vi "CFocus.vi"() -> ()   [LabVIEW 2012]
uses:
  Madlib.dll
panel:
  in  "Read Rate":bool=TRUE
  in  "Stream Rate":i32(slide)=100 min=100 max=1000 step=1 scale=100.0..1000.0 scale format="%#.0f"
  out "resetProgress":u8(slide) scale=0.0..100.0
  in  "resetEncoder":bool
  out "Graph":T1(graph)
  in  "C-Focus":bool
  out "MCL_Error":i32
  out "Tab Control":enum32{"Position Control", "C-Focus Control"}(tab)
  in  "Position":dbl
  in  "Command":bool
  in  "Start":dbl min=0.0
  in  "End":dbl min=0.0
  in  "# of Steps":dbl=1.0 min=1.0
  in  "Dwell Time":u32
  out "Calculated Step Size":dbl
  in  "Z-Stack":bool
  in  "Relative position\nchange from current":dbl step=0.005
  in  "CF command":bool
  out "Enabled at (ADC)":dbl format="%#.4f"
  in  "Z-Stack with C-Focus":bool
  in  "Dwell Time 2":u32
  in  "# of Steps 2":dbl=1.0 min=1.0
  out "End 2":dbl min=0.0 format="%#.4f"
  out "Start 2":dbl min=0.0 format="%#.4f"
  in  "Step Size":dbl step=0.005
  out "EncoderStart":dbl
  out "Error":i32
  in  "EndVI":bool
  out "Mode Bar":enum32{"Standard", "Cfocus"}(tab)
  # "Enable/Disable Constant Focus"
  # "Stream\nRate"
  # "Read\nRate"
  # "fast"
  # "slow"
  # "fast"
  # "slow"
  # "Positioning"
  # "um"
  # "Z-Stack"
  # "um"
  # "um"
  # "ms"
  # "um"
  # "Position Info"
  # "um"
  # "C-Focus Positioning"
  # "um"
  # "C-Focus Z-Stack"
  # "um"
  # "ms"
  # "um"
  # "um"
  # "Standard Position Control"
  # "Constant Focus Mode Enabled"
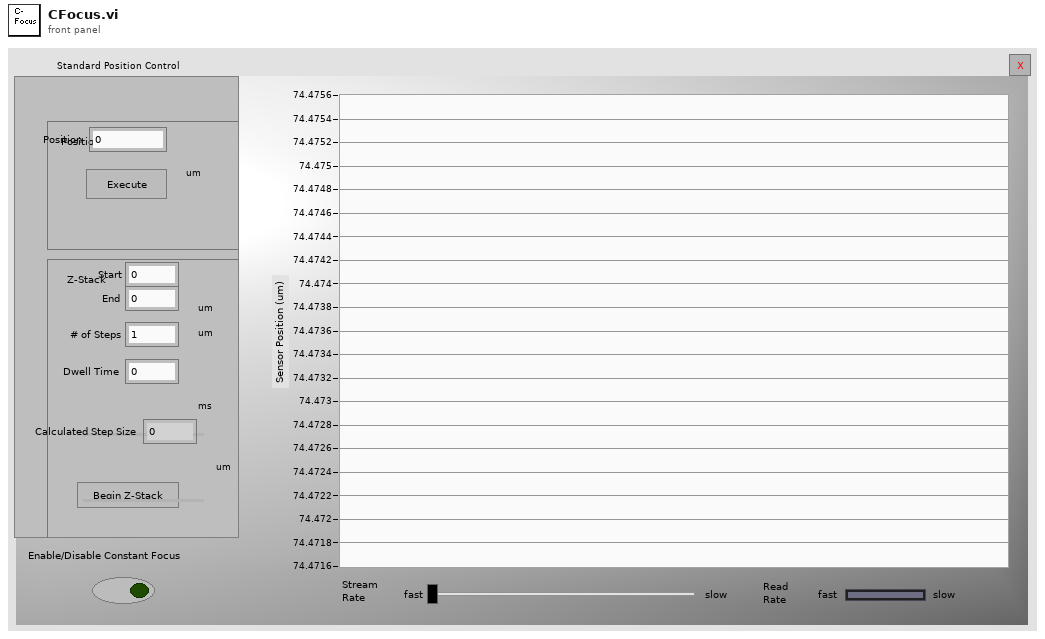
[diagram p1: front panel]
types:
  T1 = cluster{"Encoder Set":dbl, "Encoder Set":dbl, dbl[][]}
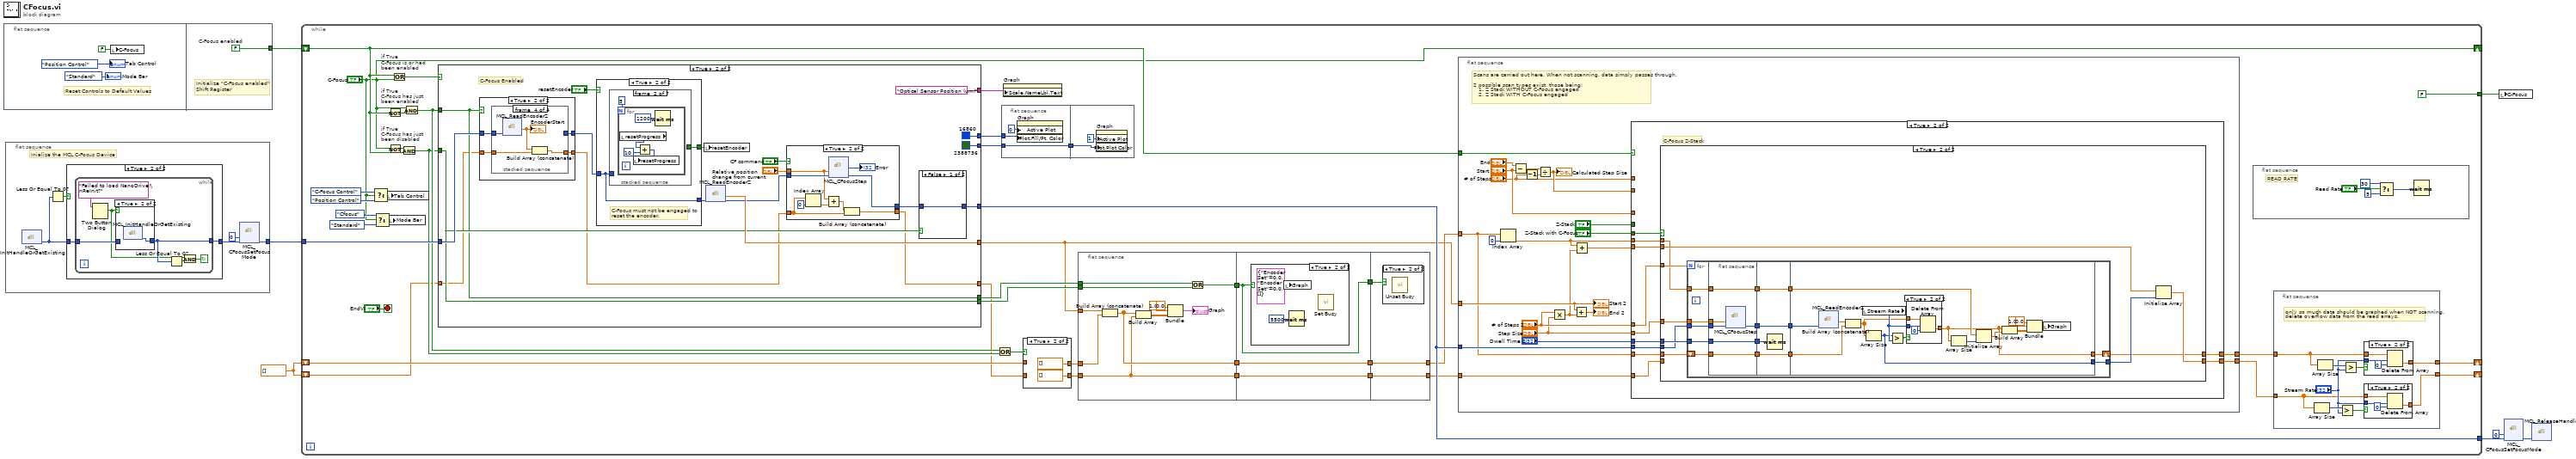
[diagram p0: block diagram]
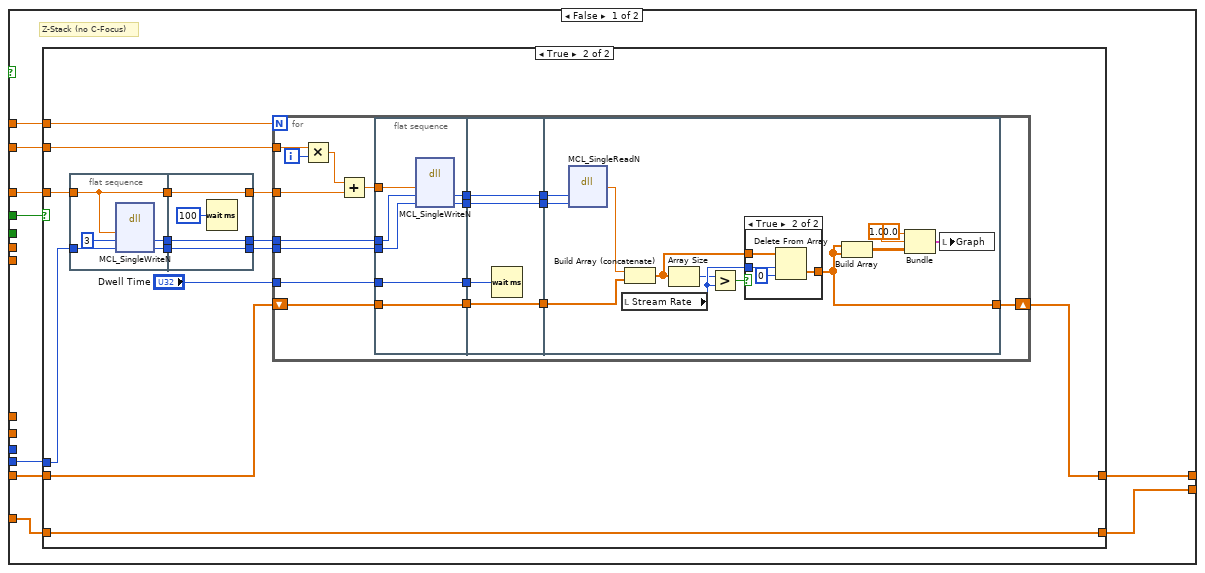
[diagram p4: hidden frame]
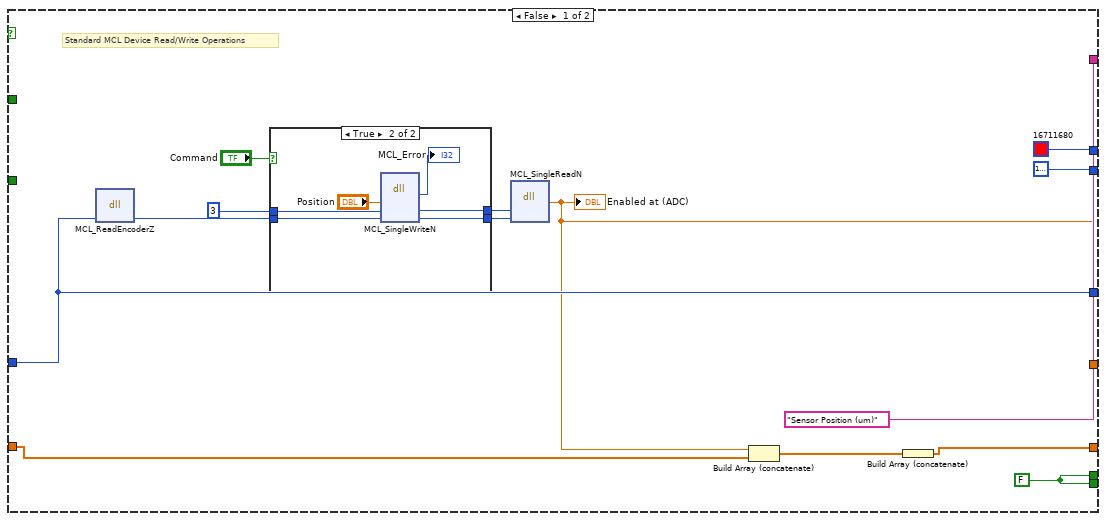
[diagram p14: hidden frame]
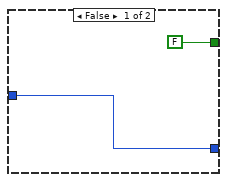
[diagram p16: hidden frame]
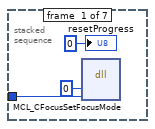
[diagram p17: hidden frame]
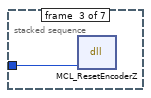
[diagram p18: hidden frame]
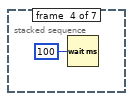
[diagram p19: hidden frame]
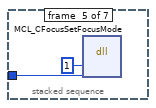
[diagram p20: hidden frame]
diagram:
  w1 = dbl[] []
  n1 = flat-sequence {
    tunnel: [w11] -> w2
    frame #0 {
      # "Reset Controls to Default Values"
      n2 = local write "C-Focus"(FALSE ("C-Focus")) -> ()
      "Tab Control" <- enum32{"Position Control", "C-Focus Control"}."Position Control" ("Tab Control")
      "Mode Bar" <- enum32{"Standard", "Cfocus"}."Standard" ("Mode Bar")
    }
    frame #1 {
      w11 = FALSE  # C-Focus enabled
      # "Initialize \"C-Focus enabled\"\nShift Register"
    }
  }
  n3 = flat-sequence {
    tunnel: [w12] -> w6
    frame #0 {
      # "Inialize the MCL C-Focus Device"
      n4 = dll-call lib="C:/Users/Labview/Desktop/SRR/Madlib_x64/Labview Examples/Madlib.dll" fn="MCL_InitHandleOrGetExisting"() -> ("return type"=w15:i32)  [unwired: 3 in, 2 out]
      n5 = Less Or Equal To 0?(x=w15) -> (x <= 0?=w16:bool)
      n6 = case shown="True" w16 {
        tunnel: w15 -> [w17 w19]
        tunnel: [w17 w18] -> w13
        frame False {
        }
        frame True {
          n7 = while {
            tunnel: w19 -> [w24]
            tunnel: [w22] -> w18
            stop <- w21 continue-if-true
            n8 = Two Button Dialog(message="Failed to load NanoDrive!\nReInit?") -> (T button?=w20:bool)  [unwired: 2 out]
            n9 = case shown="True" w20 {
              tunnel: w24 -> [w26 _]
              tunnel: [w26 w27] -> w22
              frame False {
              }
              frame True {
                n10 = dll-call lib="C:/Users/Labview/Desktop/SRR/Madlib_x64/Labview Examples/Madlib.dll" fn="MCL_InitHandleOrGetExisting"() -> ("return type"=w27:i32)  [unwired: 3 in, 2 out]
              }
            }
            n11 = Less Or Equal To 0?(x=w22) -> (x <= 0?=w23:bool)
            n12 = And(x=w20, y=w23) -> (x .and. y?=w21:bool)
          }
        }
      }
      n13 = dll-call lib="C:/Users/Labview/Desktop/SRR/Madlib_x64/Labview Examples/Madlib.dll" fn="MCL_CFocusSetFocusMode" ("MADLib.dll:MCL_ReadEncoderZ")("C-Focus Enable"=i16 0, "handle"=w13) -> ("handle"=w12:i32)  [unwired: 4 in, 3 out]
    }
  }
  n14 = while {
    tunnel: [w66] -> w4
    tunnel: w6 -> [w68]
    shift-right: ["C-Focus"] -> _
    shift-left: w2 -> [w64]
    tunnel: [FALSE ("C-Focus")] -> w7
    shift-right: [w42] -> _
    shift-left: w1 -> [w52]
    shift-right: [w41] -> _
    shift-left: w1 -> [w46]
    stop <- "EndVI" stop-if-true
    # "if True\nC-Focus is or had been enabled"
    # "if True\nC-Focus has just\nbeen disabled"
    # "if True\nC-Focus has just\nbeen enabled"
    n15 = Select(t=enum32{"Position Control", "C-Focus Control"}."C-Focus Control" ("Tab Control"), s="C-Focus", f=enum32{"Position Control", "C-Focus Control"}."Position Control" ("Tab Control")) -> (s? t:f=w59:enum32{"Position Control", "C-Focus Control"})
    n16 = Select(t=enum32{"Standard", "Cfocus"}."Cfocus" ("Mode Bar"), s="C-Focus", f=enum32{"Standard", "Cfocus"}."Standard" ("Mode Bar")) -> (s? t:f=w37:enum32{"Standard", "Cfocus"})
    n17 = local write "Tab Control"(w59) -> ()
    n18 = Not(x=w64) -> (.not. x?=w63:bool)
    n19 = Not(x="C-Focus") -> (.not. x?=w62:bool)
    n20 = local write "Mode Bar"(w37) -> ()
    n21 = Or(x=w64, y="C-Focus") -> (x .or. y?=w65:bool)
    n22 = And(x=w62, y=w64) -> (x .and. y?=w47:bool)
    n23 = And(x="C-Focus", y=w63) -> (x .and. y?=w49:bool)
    n24 = case shown="True" w65 {
      tunnel: [w300 w331] -> w66
      tunnel: w68 -> [w300 w328]
      tunnel: w49 -> [_ w317]
      tunnel: w47 -> [_ w318]
      tunnel: [w295 w329] -> w28
      tunnel: [u32 16711680 u32 16860] -> w54
      tunnel: ["Sensor Position (um)" ("Y Scale.Unit Label.Text") "Optical Sensor Position (um)" ("Y Scale.Unit Label.Text")] -> w53
      tunnel: [w297 w318] -> w57
      tunnel: [w297 w317] -> w56
      tunnel: w46 -> [w291 w315]
      tunnel: [w294 w316] -> w45
      tunnel: [u32 16777216 u32 2388736] -> w43
      frame False {
        w297 = FALSE
        # "Standard MCL Device Read/Write Operations"
        n25 = dll-call lib="C:/Users/Labview/Desktop/SRR/Madlib_x64/Labview Examples/Madlib.dll" fn="MCL_ReadEncoderZ"("handle"=w300) -> ("handle"=w296:i32)  [unwired: 3 in, 3 out]
        n26 = case shown="True" "Command" {
          tunnel: w296 -> [w306 w312]
          tunnel: [w306 w311] -> w304
          tunnel: [w305 w310] -> w303
          tunnel: 3 ("axis") -> [w305 w308]
          frame False {
          }
          frame True {
            n27 = dll-call lib="C:/Users/Labview/Desktop/SRR/Madlib_x64/Labview Examples/Madlib.dll" fn="MCL_SingleWriteN"("Position"="Position", "axis"=w308, "handle"=w312) -> ("MCL_Error"=→"MCL_Error":i32, "axis"=w310:i32, "handle"=w311:i32)  [unwired: 4 in, 2 out]
          }
        }
        n28 = dll-call lib="C:/Users/Labview/Desktop/SRR/Madlib_x64/Labview Examples/Madlib.dll" fn="MCL_SingleReadN"("axis"=w303, "handle"=w304) -> ("Position Read"=w295:dbl)  [unwired: 5 in, 2 out]
        "Enabled at (ADC)" <- w295
        n29 = Build Array (concatenate)(w295, w291) -> (w292:dbl[])
        n30 = Build Array (concatenate)(w292) -> (w294:dbl[])
      }
      frame True {
        # "C-Focus Enabled"
        n31 = case shown="True" w317 {
          tunnel: w328 -> [w360 w364]
          tunnel: [w360 w363] -> w324
          tunnel: w315 -> [w359 w362]
          tunnel: [w359 w361] -> w314
          frame False {
          }
          frame True {
            n32 = stacked-sequence {
              tunnel: w364 -> [w365 w368 _ w373]
              tunnel: [_ w366 _ _] -> w363
              tunnel: w362 -> [_ _ _ w372]
              tunnel: [_ _ _ w371] -> w361
              frame #0 {
                # "reset"
                n33 = dll-call lib="C:/Users/Labview/Desktop/SRR/Madlib_x64/Labview Examples/Madlib.dll" fn="MCL_ResetEncoderZ" ("MADLib.dll:MCL_ReadEncoderZ")("handle"=w365) -> ()  [unwired: 4 in, 3 out]
              }
              frame #1 {
                # "engage"
                n34 = dll-call lib="C:/Users/Labview/Desktop/SRR/Madlib_x64/Labview Examples/Madlib.dll" fn="MCL_CFocusSetFocusMode" ("MADLib.dll:MCL_ReadEncoderZ")("C-Focus Enable"=i16 1, "handle"=w368) -> ("handle"=w366:i32)  [unwired: 4 in, 3 out]
              }
              frame #2 {
                n35 = Wait (ms)(milliseconds to wait=u32 100) -> ()  [unwired: 1 out]
              }
              frame #3 {
                n36 = dll-call lib="C:/Users/Labview/Desktop/SRR/Madlib_x64/Labview Examples/Madlib.dll" fn="MCL_ReadEncoderZ"("handle"=w373) -> ("Encoder Read"=w370:dbl)  [unwired: 4 in, 2 out]
                "EncoderStart" <- w370
                n37 = Build Array (concatenate)(w370, w372) -> (w371:dbl[])
              }
            }
          }
        }
        n38 = case shown="True" "resetEncoder" {
          tunnel: w324 -> [w333 w335]
          tunnel: [w333 w335] -> w323
          tunnel: [FALSE ("resetEncoder") w334] -> w321
          frame False {
          }
          frame True {
            # "C-Focus must not be engaged to\nreset the encoder."
            n39 = stacked-sequence {
              tunnel: w335 -> [w337 _ w344 _ w346 _ w353]
              tunnel: [_ _ _ _ _ _ FALSE ("resetEncoder")] -> w334
              frame #0 {
                n40 = dll-call lib="C:/Users/Labview/Desktop/SRR/Madlib_x64/Labview Examples/Madlib.dll" fn="MCL_CFocusSetFocusMode" ("MADLib.dll:MCL_ReadEncoderZ")("C-Focus Enable"=i16 0, "handle"=w337) -> ()  [unwired: 5 in, 3 out]
                "resetProgress" <- u8 0 ("resetProgress")
              }
              frame #1 {
                n41 = for {
                  N: 5 -> [_]
                  n42 = local read "resetProgress"() -> (w342:u8)
                  n43 = Add(x=w342, y=u8 10) -> (x+y=w341:u8)
                  n44 = local write "resetProgress"(w341) -> ()
                  n45 = Wait (ms)(milliseconds to wait=u32 1200) -> ()  [unwired: 1 out]
                }
              }
              frame #2 {
                n46 = dll-call lib="C:/Users/Labview/Desktop/SRR/Madlib_x64/Labview Examples/Madlib.dll" fn="MCL_ResetEncoderZ" ("MADLib.dll:MCL_ReadEncoderZ")("handle"=w344) -> ()  [unwired: 4 in, 3 out]
              }
              frame #3 {
                n47 = Wait (ms)(milliseconds to wait=u32 100) -> ()  [unwired: 1 out]
              }
              frame #4 {
                n48 = dll-call lib="C:/Users/Labview/Desktop/SRR/Madlib_x64/Labview Examples/Madlib.dll" fn="MCL_CFocusSetFocusMode" ("MADLib.dll:MCL_ReadEncoderZ")("C-Focus Enable"=i16 1, "handle"=w346) -> ()  [unwired: 5 in, 3 out]
              }
              frame #5 {
                n49 = local read "resetProgress"() -> (w349:u8)
                n50 = Add(x=w349, y=u8 30) -> (x+y=w348:u8)
                n51 = local write "resetProgress"(w348) -> ()
                n52 = Wait (ms)(milliseconds to wait=u32 5100) -> ()  [unwired: 1 out]
              }
              frame #6 {
                n53 = dll-call lib="C:/Users/Labview/Desktop/SRR/Madlib_x64/Labview Examples/Madlib.dll" fn="MCL_ReadEncoderZ"("handle"=w353) -> ("Encoder Read"=w354:dbl)  [unwired: 4 in, 2 out]
                n54 = local write "EncoderStart"(w354) -> ()
              }
            }
          }
        }
        n55 = local write "resetEncoder"(w321) -> ()
        n56 = dll-call lib="C:/Users/Labview/Desktop/SRR/Madlib_x64/Labview Examples/Madlib.dll" fn="MCL_ReadEncoderZ"("handle"=w323) -> ("Encoder Read"=w329:dbl, "handle"=w327:i32)  [unwired: 3 in, 2 out]
        n57 = case shown="True" "CF command" {
          tunnel: w327 -> [w378 w381]
          tunnel: "Relative position\nchange from current" -> [_ w379]
          tunnel: [w378 w387] -> w325
          tunnel: w314 -> [w374 w384]
          tunnel: [w376 w380] -> w316
          frame False {
            n58 = Index Array(array=w374, index=0) -> (element=w375:dbl)
            n59 = Build Array (concatenate)(w375, w374) -> (w376:dbl[])
          }
          frame True {
            n60 = Index Array(array=w384, index=0) -> (element=w382:dbl)
            n61 = Add(x=w379, y=w382) -> (x+y=w383:dbl)
            n62 = dll-call lib="C:/Users/Labview/Desktop/SRR/Madlib_x64/Labview Examples/Madlib.dll" fn="MCL_CFocusStep"("arg1"=w379, "handle"=w381) -> ("return type"=→"Error":i32, "handle"=w387:i32)  [unwired: 4 in, 2 out]
            n63 = Build Array (concatenate)(w383, w384) -> (w380:dbl[])
          }
        }
        n64 = case shown="False" w318 {
          tunnel: [w355 w358] -> w331
          tunnel: w325 -> [w355 w357]
          frame False {
          }
          frame True {
            n65 = dll-call lib="C:/Users/Labview/Desktop/SRR/Madlib_x64/Labview Examples/Madlib.dll" fn="MCL_CFocusSetFocusMode" ("MADLib.dll:MCL_ReadEncoderZ")("C-Focus Enable"=i16 0, "handle"=w357) -> ("handle"=w358:i32)  [unwired: 4 in, 3 out]
          }
        }
      }
    }
    n66 = Or(x=w49, y=w47) -> (x .or. y?=w48:bool)
    n67 = flat-sequence {
      tunnel: w54 -> [w265]
      tunnel: [w263] -> w44
      tunnel: w43 -> [w263]
      tunnel: w44 -> [w266]
      frame #0 {
        n68 = property on="Graph" class="WFGraph (strict)"("Active Plot"=u32 0, "Plot.Fill/Pt. Color"=w265) -> ()  [unwired: 2 in, 2 out]
      }
      frame #1 {
        n69 = property on="Graph" class="WFGraph (strict)"("Active Plot"=u32 1, "Plot.Plot Color"=w266) -> ()  [unwired: 2 in, 2 out]
      }
    }
    n70 = property on="Graph" class="WFGraph (strict)"("YScale.NameLbl.Text"=w53) -> ()  [unwired: 2 in, 2 out]
    n71 = case shown="True" w48 {
      tunnel: w52 -> [w269 _]
      tunnel: [w269 dbl[] []] -> w51
      tunnel: w45 -> [w268 _]
      tunnel: [w268 dbl[] []] -> w50
      frame False {
      }
      frame True {
      }
    }
    n72 = flat-sequence {
      tunnel: w28 -> [w282]
      tunnel: [w280] -> w58
      tunnel: w57 -> [w281]
      tunnel: w56 -> [w279]
      tunnel: w51 -> [w274]
      tunnel: w50 -> [w272]
      tunnel: [w273] -> w35
      tunnel: [w272] -> w33
      tunnel: w58 -> [w285]
      tunnel: [w285] -> w55
      tunnel: [w284] -> w36
      tunnel: w35 -> [w284]
      tunnel: [w283] -> w34
      tunnel: w33 -> [w283]
      tunnel: w55 -> [w290]
      tunnel: [w289] -> w32
      tunnel: w36 -> [w289]
      tunnel: [w288] -> w31
      tunnel: w34 -> [w288]
      frame #0 {
        n73 = Build Array (concatenate)(w282, w274) -> (w273:dbl[])
        n74 = Build Array(w273, w272) -> (w276:dbl[][])
        n75 = Bundle("Encoder Set"=0.0, "Encoder Set"=1.0, w276) -> (→"Graph":T1)  [unwired: 1 out]
        n76 = Or(x=w279, y=w281) -> (x .or. y?=w280:bool)
      }
      frame #1 {
        n77 = case shown="True" w285 {
          frame False {
          }
          frame True {
            n78 = local write "Graph"(T1 {"Encoder Set"=0.0, "Encoder Set"=0.0, []} ("Graph")) -> ()
            n79 = Wait (ms)(milliseconds to wait=u32 5500) -> ()  [unwired: 1 out]
            n80 = call <vilib>:"Set Busy.vi"() -> ()  [unwired: 4 in, 8 out]
          }
        }
      }
      frame #2 {
        n81 = case shown="True" w290 {
          frame False {
          }
          frame True {
            n82 = call <vilib>:"Unset Busy.vi"() -> ()  [unwired: 2 in, 10 out]
          }
        }
      }
    }
    n83 = flat-sequence {
      tunnel: w66 -> [w92]
      tunnel: w64 -> [w91]
      tunnel: w28 -> [w81]
      tunnel: w32 -> [w75]
      tunnel: w31 -> [w74]
      tunnel: [w73] -> w30
      tunnel: [w72] -> w29
      frame #0 {
        # "Scans are carried out here. When not scanning, data simply passes through.\n\n2 possible scan types exist, those being:\n   1. Z Stack WITHOUT C-Focus engaged\n   2. Z Stack WITH C-Focus engaged"
        n84 = Index Array(array=w75, index=0) -> (element=w78:dbl)
        n85 = Subtract(x="End", y="Start") -> (x-y=w90:dbl)
        n86 = Decrement(x="# of Steps") -> (x-1=w71:dbl)
        n87 = Divide(x=w90, y=w71) -> (x/y=w87:dbl)
        "Calculated Step Size" <- w87
        n88 = Multiply(x="# of Steps 2", y="Step Size") -> (x*y=w76:dbl)
        n89 = Add(x=w81, y=w76) -> (x+y=→"End 2":dbl)
        n90 = Add(x=w78, y=w76) -> (x+y=w77:dbl)
        n91 = case shown="True" w91 {
          tunnel: w92 -> [w101 w179]
          tunnel: "# of Steps" -> [w100 _]
          tunnel: "Start" -> [w99 _]
          tunnel: w87 -> [w98 _]
          tunnel: "Z-Stack" -> [w97 _]
          tunnel: "Dwell Time 2" -> [_ w183]
          tunnel: "# of Steps 2" -> [_ w182]
          tunnel: "Step Size" -> [_ w181]
          tunnel: "Z-Stack with C-Focus" -> [_ w180]
          tunnel: w75 -> [w93 w178]
          tunnel: w74 -> [w95 w177]
          tunnel: [w94 w176] -> w72
          tunnel: [w96 w175] -> w73
          tunnel: w78 -> [_ w174]
          tunnel: w77 -> [_ w173]
          frame False {
            # "Z-Stack (no C-Focus)"
            n92 = case shown="True" w97 {
              tunnel: w101 -> [_ w107]
              tunnel: w100 -> [_ w110]
              tunnel: w99 -> [_ w109]
              tunnel: w98 -> [_ w108]
              tunnel: [w103 w106] -> w96
              tunnel: w95 -> [w103 w106]
              tunnel: [w102 w104] -> w94
              tunnel: w93 -> [w102 w105]
              frame False {
              }
              frame True {
                n93 = flat-sequence {
                  tunnel: w109 -> [w120]
                  tunnel: w107 -> [w122]
                  tunnel: [w120] -> w117
                  tunnel: [w119] -> w116
                  tunnel: [w118] -> w115
                  tunnel: [w125] -> w113
                  tunnel: w117 -> [w125]
                  tunnel: w116 -> [w124]
                  tunnel: w115 -> [w123]
                  tunnel: [w124] -> w112
                  tunnel: [w123] -> w111
                  frame #0 {
                    n94 = dll-call lib="C:/Users/Labview/Desktop/SRR/Madlib_x64/Labview Examples/Madlib.dll" fn="MCL_SingleWriteN" ("MADLib.dll:MCL_CFocusStep")("Position"=w120, "axis"=3, "handle"=w122) -> ("axis"=w119:i32, "handle"=w118:i32)  [unwired: 4 in, 3 out]
                  }
                  frame #1 {
                    n95 = Wait (ms)(milliseconds to wait=u32 100) -> ()  [unwired: 1 out]
                  }
                }
                n96 = for {
                  N: w110 -> [_]
                  tunnel: "Dwell Time" -> [w136]
                  tunnel: w113 -> [w140]
                  tunnel: w112 -> [w138]
                  tunnel: w111 -> [w137]
                  tunnel: w108 -> [w142]
                  shift-right: [w127] -> w104
                  shift-left: w105 -> [w131]
                  i -> [w143]
                  n97 = Multiply(x=w142, y=w143) -> (x*y=w141:dbl)
                  n98 = Add(x=w141, y=w140) -> (x+y=w139:dbl)
                  n99 = flat-sequence {
                    tunnel: w139 -> [w150]
                    tunnel: w138 -> [w149]
                    tunnel: w137 -> [w148]
                    tunnel: w136 -> [w145]
                    tunnel: [w147] -> w135
                    tunnel: [w146] -> w134
                    tunnel: [w145] -> w133
                    tunnel: [w144] -> w132
                    tunnel: w131 -> [w144]
                    tunnel: w135 -> [w154]
                    tunnel: w134 -> [w153]
                    tunnel: w133 -> [w152]
                    tunnel: w132 -> [w151]
                    tunnel: [w154] -> w130
                    tunnel: [w153] -> w129
                    tunnel: [w151] -> w128
                    tunnel: w130 -> [w156]
                    tunnel: w129 -> [w155]
                    tunnel: w128 -> [w158]
                    tunnel: [w157] -> w127
                    frame #0 {
                      n100 = dll-call lib="C:/Users/Labview/Desktop/SRR/Madlib_x64/Labview Examples/Madlib.dll" fn="MCL_SingleWriteN" ("MADLib.dll:MCL_CFocusStep")("Position"=w150, "axis"=w149, "handle"=w148) -> ("axis"=w147:i32, "handle"=w146:i32)  [unwired: 4 in, 3 out]
                    }
                    frame #1 {
                      n101 = Wait (ms)(milliseconds to wait=w152) -> ()  [unwired: 1 out]
                    }
                    frame #2 {
                      n102 = dll-call lib="C:/Users/Labview/Desktop/SRR/Madlib_x64/Labview Examples/Madlib.dll" fn="MCL_SingleReadN" ("MADLib.dll:MCL_CFocusStep")("axis"=w156, "handle"=w155) -> ("Position Read"=w159:dbl)  [unwired: 5 in, 2 out]
                      n103 = local read "Stream Rate"() -> (w167:i32)
                      n104 = Build Array (concatenate)(w159, w158) -> (w166:dbl[])
                      n105 = Array Size(array=w166) -> (size(s)=w163:i32)
                      n106 = Greater?(x=w163, y=w167) -> (0:w165:bool)
                      n107 = case shown="True" w165 {
                        tunnel: w166 -> [w168 w172]
                        tunnel: [w168 w169] -> w157
                        tunnel: w167 -> [_ w170]
                        frame False {
                        }
                        frame True {
                          n108 = Delete From Array(array=w172, length=w170, index=0) -> (deleted portion=w169:dbl[])  [unwired: 1 out]
                        }
                      }
                      n109 = Build Array(w157, w157) -> (w162:dbl[][])
                      n110 = Bundle("Encoder Set"=0.0, "Encoder Set"=1.0, w162) -> (w164:T1)  [unwired: 1 out]
                      n111 = local write "Graph"(w164) -> ()
                    }
                  }
                }
              }
            }
          }
          frame True {
            # "C-Focus Z-Stack"
            n112 = case shown="True" w180 {
              tunnel: w183 -> [_ w195]
              tunnel: w182 -> [_ w194]
              tunnel: w181 -> [_ w193]
              tunnel: w179 -> [_ w192]
              tunnel: w178 -> [w184 w189]
              tunnel: w177 -> [w185 _]
              tunnel: [w184 w186] -> w176
              tunnel: [w185 w190] -> w175
              tunnel: w174 -> [_ w187]
              tunnel: w173 -> [_ w191]
              frame False {
              }
              frame True {
                n113 = for {
                  N: w194 -> [_]
                  tunnel: w195 -> [w209]
                  tunnel: w193 -> [w207]
                  tunnel: w192 -> [w208]
                  tunnel: [w200] -> w188
                  tunnel: w187 -> [w199]
                  shift-right: [w196] -> w186
                  shift-left: w189 -> [w201]
                  n114 = flat-sequence {
                    tunnel: w209 -> [w214]
                    tunnel: w208 -> [w215]
                    tunnel: w207 -> [w212]
                    tunnel: [w214] -> w206
                    tunnel: [w213] -> w205
                    tunnel: [w211] -> w202
                    tunnel: w201 -> [w211]
                    tunnel: w199 -> [w210]
                    tunnel: [w210] -> w197
                    tunnel: w206 -> [w218]
                    tunnel: w205 -> [w219]
                    tunnel: [w219] -> w204
                    tunnel: [w217] -> w203
                    tunnel: w202 -> [w217]
                    tunnel: [w216] -> w198
                    tunnel: w197 -> [w216]
                    tunnel: w204 -> [w224]
                    tunnel: w203 -> [w223]
                    tunnel: [w222] -> w200
                    tunnel: w198 -> [w221]
                    tunnel: [w220] -> w196
                    frame #0 {
                      n115 = dll-call lib="C:/Users/Labview/Desktop/SRR/Madlib_x64/Labview Examples/Madlib.dll" fn="MCL_CFocusStep"("arg1"=w212, "handle"=w215) -> ("handle"=w213:i32)  [unwired: 4 in, 3 out]
                    }
                    frame #1 {
                      n116 = Wait (ms)(milliseconds to wait=w218) -> ()  [unwired: 1 out]
                    }
                    frame #2 {
                      n117 = dll-call lib="C:/Users/Labview/Desktop/SRR/Madlib_x64/Labview Examples/Madlib.dll" fn="MCL_ReadEncoderZ"("handle"=w224) -> ("Encoder Read"=w226:dbl)  [unwired: 4 in, 2 out]
                      n118 = Build Array (concatenate)(w226, w223) -> (w227:dbl[])
                      n119 = local read "Stream Rate"() -> (w234:i32)
                      n120 = Array Size(array=w227) -> (size(s)=w222:i32)
                      n121 = Greater?(x=w222, y=w234) -> (0:w225:bool)
                      n122 = case shown="True" w225 {
                        tunnel: w227 -> [w235 w239]
                        tunnel: [w235 w236] -> w220
                        tunnel: w234 -> [_ w237]
                        frame False {
                        }
                        frame True {
                          n123 = Delete From Array(array=w239, length=w237, index=0) -> (deleted portion=w236:dbl[])  [unwired: 1 out]
                        }
                      }
                      n124 = Array Size(array=w220) -> (size(s)=w233:i32)
                      n125 = Initialize Array(w221, w233) -> (w232:dbl[])
                      n126 = Build Array(w220, w232) -> (w231:dbl[][])
                      n127 = Bundle("Encoder Set"=0.0, "Encoder Set"=1.0, w231) -> (w230:T1)  [unwired: 1 out]
                      n128 = local write "Graph"(w230) -> ()
                    }
                  }
                }
                n129 = Initialize Array(w191, w188) -> (w190:dbl[])
              }
            }
          }
        }
        "Start 2" <- w81
      }
    }
    n130 = flat-sequence {
      frame #0 {
        # "READ RATE"
        n131 = Select(t=u32 30 ("y"), s="Read Rate", f=u32 5) -> (s? t:f=w260:u32)
        n132 = Wait (ms)(milliseconds to wait=w260) -> ()  [unwired: 1 out]
      }
    }
    n133 = flat-sequence {
      tunnel: [w245] -> w42
      tunnel: [w242] -> w41
      tunnel: w30 -> [w241]
      tunnel: w29 -> [w240]
      frame #0 {
        # "only so much data should be graphed when NOT scanning.\ndelete overflow data from the read arrays."
        n134 = Array Size(array=w241) -> (size(s)=w247:i32)
        n135 = Array Size(array=w240) -> (size(s)=w248:i32)
        n136 = Greater?(x=w247, y="Stream Rate") -> (0:w244:bool)
        n137 = Greater?(x=w248, y="Stream Rate") -> (0:w246:bool)
        n138 = case shown="True" w244 {
          tunnel: w241 -> [w249 w253]
          tunnel: [w249 w250] -> w242
          tunnel: "Stream Rate" -> [_ w251]
          frame False {
          }
          frame True {
            n139 = Delete From Array(array=w253, length=w251, index=0) -> (deleted portion=w250:dbl[])  [unwired: 1 out]
          }
        }
        n140 = case shown="True" w246 {
          tunnel: w240 -> [w254 w258]
          tunnel: [w254 w255] -> w245
          tunnel: "Stream Rate" -> [_ w256]
          frame False {
          }
          frame True {
            n141 = Delete From Array(array=w258, length=w256, index=0) -> (deleted portion=w255:dbl[])  [unwired: 1 out]
          }
        }
      }
    }
  }
  n142 = local write "C-Focus"(w7) -> ()
  n143 = dll-call lib="C:/Users/Labview/Desktop/SRR/Madlib_x64/Labview Examples/Madlib.dll" fn="MCL_CFocusSetFocusMode" ("MADLib.dll:MCL_ReadEncoderZ")("C-Focus Enable"=i16 0, "handle"=w4) -> ("handle"=w3:i32)  [unwired: 4 in, 3 out]
  n144 = dll-call lib="C:/Users/Labview/Desktop/SRR/Madlib_x64/Labview Examples/Madlib.dll" fn="MCL_ReleaseHandle"("handle"=w3) -> ()  [unwired: 4 in, 3 out]
